vi "Read Homed.vi"(8 "error in (no error)":errorcluster, 11 "XY Stage Data Class in":refnum<class "XY Stage Data Class.lvclass">) -> (0 "error out":errorcluster, 2 "Homed":T1, 3 "XY Stage Data Class out":refnum<class "XY Stage Data Class.lvclass">)   [LabVIEW 2022 SP3, in "XY Stage Data Class.lvclass"]
uses:
  XY Stage Data Class.lvclass
  XY Stage Data Class.lvclass/XY Stage Data Class.ctl
  Homed.ctl
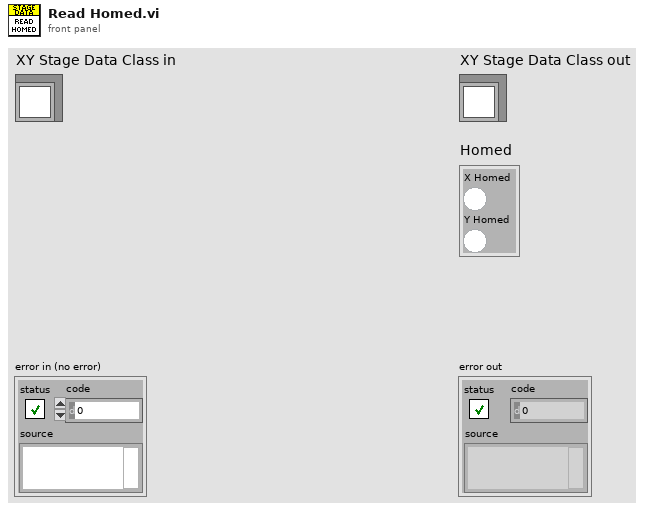
[diagram p1: front panel]
types:
  T1 = typedef "XY Stage Data Class.lvclass/Homed.ctl" = cluster{"X Homed":bool, "Y Homed":bool}
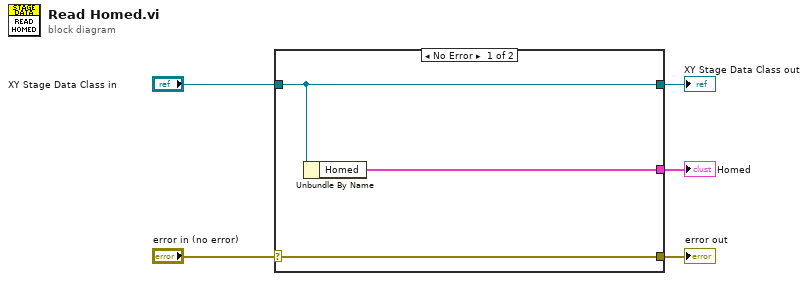
[diagram p0: block diagram]
diagram:
  n1 = case shown="No Error" "error in (no error)" {
    selector: "error in (no error)" -> [w8 w9]
    tunnel: [w8 w9] -> w4
    tunnel: [w7 w10] -> w2
    tunnel: "XY Stage Data Class in" -> [w7 w10]
    tunnel: [w6 _] -> w1
    frame No Error {
      n2 = Unbundle By Name(w7) -> ("Homed"=w6:T1)
    }
    frame Error {
    }
  }
  "error out" <- w4
  "XY Stage Data Class out" <- w2
  "Homed" <- w1
